vi "getIVSweepResults.vi"(8 "error in (no error)":errorcluster, 11 "Instrument.Lockin in":refnum<class "Instrument.Lockin.lvclass">) -> (0 "error out":errorcluster, 2 "getIVSweepResults":T1, 3 "Instrument.Lockin out":refnum<class "Instrument.Lockin.lvclass">)   [LabVIEW 2016, in "Instrument.Lockin.lvclass"]
doc: "API to get the results of lockin calculation.\n\nIf address=\"\", this API reads from localhost\nIf address is remote lockin, you need to add this computer to allowed whitelist on the lockin computer you are trying to access."
uses:
  Instrument.Lockin.lvclass
  Instrument.Lockinl.UI/Typedefs/Lockin.Commands--Enum.ctl
  LockinDAQ/Typedefs/PublicEvents--LockinDAQ.getIVSweepResults.ctl
  LockinDAQ/LockinDAQ.lvclass
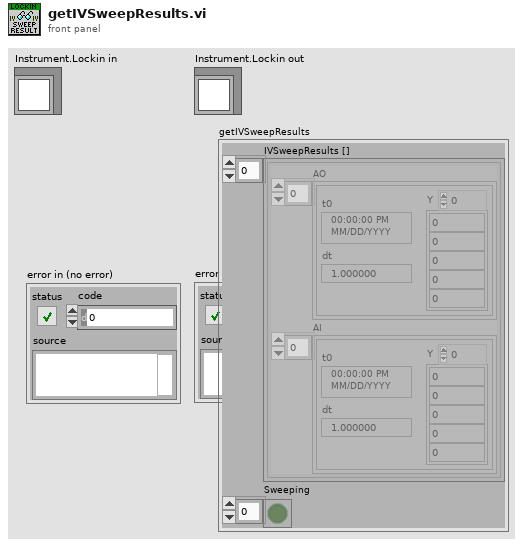
[diagram p1: front panel]
types:
  T1 = typedef "LockinDAQ.lvclass/PublicEvents--LockinDAQ.getIVSweepResults.ctl" = cluster{"IVSweepResults []":cluster{"AO":waveform(dbl)[], "AI":waveform(dbl)[]}[], "Sweeping":bool[]}
  T2 = typedef "Instrument.Lockin.lvclass/Lockin.Commands--Enum.ctl" = enum16{"setAO", "setAO_Amplitude", "setAO_DC", "setAO_Frequency", "setAO_Phase", "setAO_Function", "setAO_I+", "setREF", "setREF_Frequency", "setREF_Phase", "setIVmode", "setAIDAQ", "setAODAQ", "Reset", "setSampling", "Trigger", "getAO", "getAI", "getResults", "getTrigger", "getIVmode", "getSampling", "getAOconfig", "getREFconfig", "setGain", "getGain", "setAutoSampling", "getAutoSampling", "setSweep", "getStatus", "getSweepResults", "getIVSweepResults", "startSweep", "stopSweep", "setAUX", "getAUX", "getRefreshTime"}
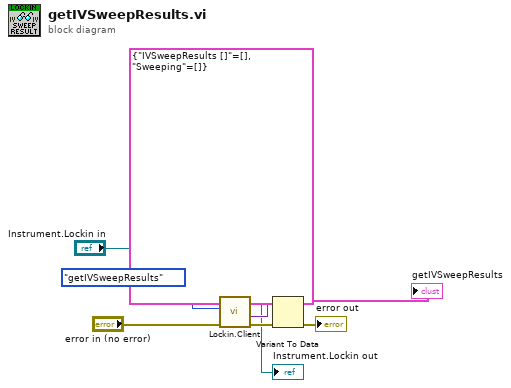
[diagram p0: block diagram]
diagram:
  n1 = call "Lockin.Client.vi"("error in (no error)"="error in (no error)", "Command"=Lockin.Commands--Enum."getIVSweepResults", "Instrument.Lockin in"="Instrument.Lockin in") -> ("error out"=w9:errorcluster, "Data out"=w8:variant, "Instrument.Lockin out"=→"Instrument.Lockin out":refnum<class "Instrument.Lockin.lvclass">)  [unwired: 6 in]
  n2 = Variant To Data(error in=w9, type=T1 {"IVSweepResults []"=[], "Sweeping"=[]} ("getIVSweepResults"), Variant=w8) -> (data=→"getIVSweepResults":T1, error out=→"error out":errorcluster)
